vi "Write connection string.vi"(8 "error in (no error)":errorcluster, 10 "connection string":string, 11 "DataSocketMessenger.lvclass in":refnum<class "DataSocketMessenger.lvclass">) -> (0 "error out":errorcluster, 3 "DataSocketMessenger.lvclass out":refnum<class "DataSocketMessenger.lvclass">)   [LabVIEW 2011, in "Messenging.lvlib" / "DataSocketMessenger.lvclass"]
uses:
  DataSocketMessenger.lvclass
  DataSocketMessenger.lvclass/DataSocketMessenger.ctl
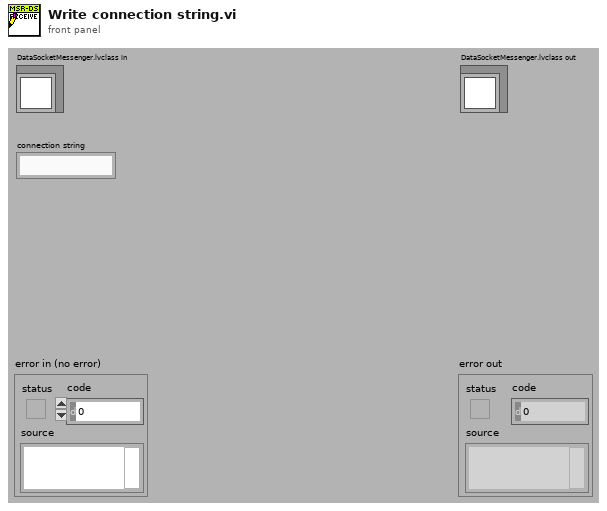
[diagram p1: front panel]
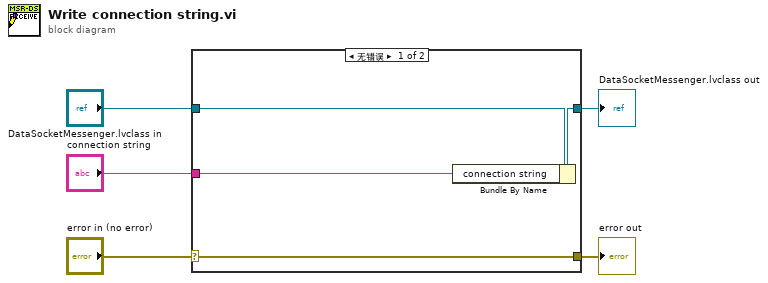
[diagram p0: block diagram]
diagram:
  n1 = case shown="无错误" "error in (no error)" {
    selector: "error in (no error)" -> [w9 w10]
    tunnel: [w9 w10] -> w4
    tunnel: [w7 w11] -> w2
    tunnel: "DataSocketMessenger.lvclass in" -> [w8 w11]
    tunnel: "connection string" -> [w6 _]
    frame No Error {
      n2 = Bundle By Name(cluster=w8, "connection string"=w6) -> (w7:refnum<class "DataSocketMessenger.lvclass">)
    }
    frame Error {
    }
  }
  "error out" <- w4
  "DataSocketMessenger.lvclass out" <- w2
